vi "Read Addr.vi"(8 "error in (no error)":errorcluster, 11 "Lakeshore 331 in":refnum<class "Lakeshore 331.lvclass">) -> (0 "error out":errorcluster, 2 "Addr":refnum<visa-resource-name>, 3 "Lakeshore 331 out":refnum<class "Lakeshore 331.lvclass">)   [LabVIEW 2022 SP3, in "Lakeshore 331.lvclass"]
uses:
  Lakeshore 331.lvclass
  Lakeshore 331.lvclass/Lakeshore 331.ctl
  Temp Control.lvclass
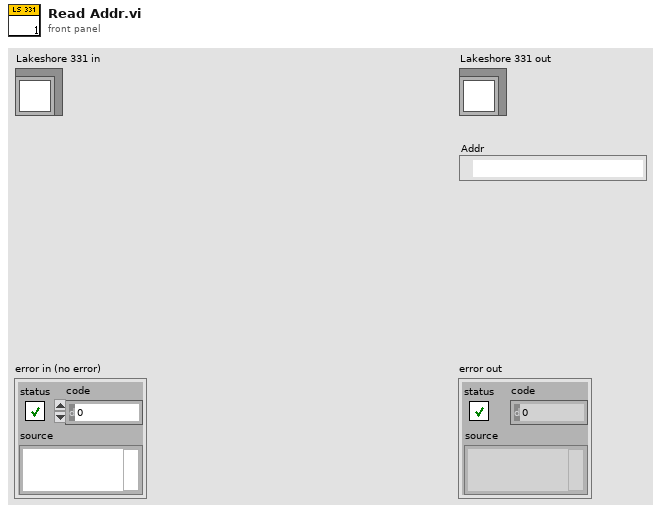
[diagram p1: front panel]
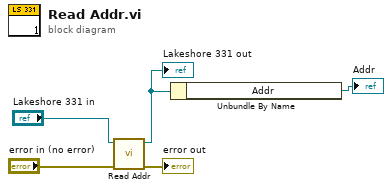
[diagram p0: block diagram]
diagram:
  n1 = call-parent "Read Addr.vi"("error in (no error)"="error in (no error)", "Temp Control in"="Lakeshore 331 in") -> ("error out"=→"error out":errorcluster, "Temp Control out"=w2:refnum<class "Lakeshore 331.lvclass">)  [unwired: 7 in, 1 out]
  "Lakeshore 331 out" <- w2
  n2 = Unbundle By Name(w2) -> ("Addr"=→"Addr":refnum<visa-resource-name>)
